vi "Create Rawdata File Name (SubVI).vi"(8 "Base Name":string="Rawdata", 12 "Output File Path":path) -> (14 "Byte Stream File out":refnum<file>)   [LabVIEW 2015]
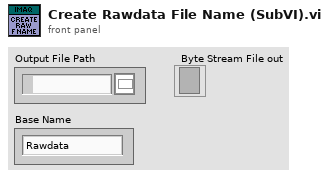
[diagram p1: front panel]
types:
  T1 = enum16{"open", "replace", "create", "open or create", "replace or create", "replace or create with confirmation"}
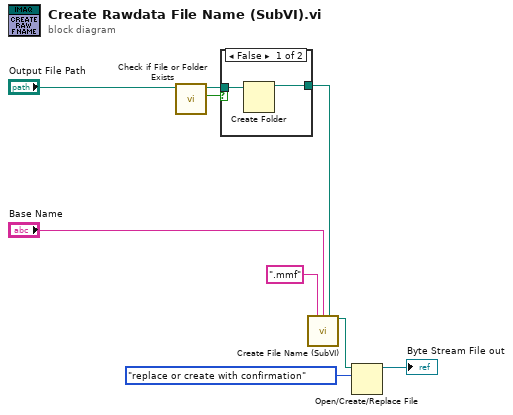
[diagram p0: block diagram]
diagram:
  n1 = call <vilib>:"Check if File or Folder Exists.vi"("path"="Output File Path") -> ("file or folder exists?"=w4:bool, "dup path"=w3:path)  [unwired: 8 in, 1 out]
  n2 = case shown="False" w4 {
    tunnel: w3 -> [w11 w12]
    tunnel: [w10 w12] -> w2
    frame False {
      n3 = Create Folder(path (use dialog)=w11) -> (created path=w10:path)  [unwired: 2 in, 2 out]
    }
    frame True {
    }
  }
  n4 = call "Create File Name (SubVI).vi"("Extension"=".mmf", "File Name Prefix"="Base Name", "File Path"=w2) -> ("File Name"=w5:path)  [unwired: 12 in]
  n5 = Open/Create/Replace File(file path (use dialog)=w5, operation (0:open)=T1."replace or create with confirmation") -> (refnum out=→"Byte Stream File out":refnum<file>)  [unwired: 4 in, 2 out]
